vi "Load Plugin From Absolute Path.vi"(2 "error in (no error)":errorcluster, 3 "Absolute Path":path) -> (0 "error out":errorcluster, 1 "Generic Plugin.lvclass":refnum<class "Generic Plugin.lvclass">)   [LabVIEW 2019, in "Generic Plugin.lvclass"]
uses:
  Generic Plugin.lvclass
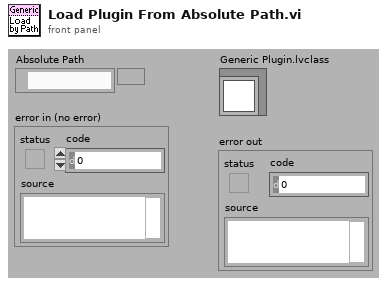
[diagram p1: front panel]
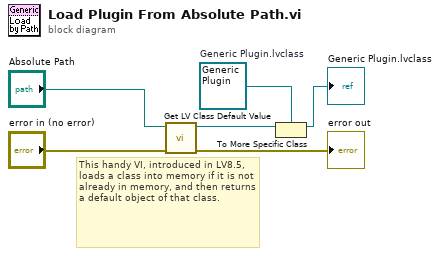
[diagram p0: block diagram]
diagram:
  w2 = refnum<class "Generic Plugin.lvclass"> refnum  # Generic Plugin.lvclass
  # "This handy VI, introduced in LV8.5, loads a class into memory if it is not already in memory, and then returns a default object of that class."
  n1 = call <vilib>:"Get LV Class Default Value.vi"("error in (no error)"="error in (no error)", "class path"="Absolute Path") -> ("error out"=→"error out":errorcluster, "object"=w4:refnum<class>)  [unwired: 8 in]
  n2 = To More Specific Class(target class=w2, reference=w4) -> (specific class reference=→"Generic Plugin.lvclass":refnum<class "Generic Plugin.lvclass">)  [unwired: 1 in, 1 out]
